vi "baseline_update.vi"(8 "current baseline phase":dbl, 9 "current baseline magnitude":dbl, 11 "Cluster in":T1={"Magnitude meas."=[], "Phase meas."=[], "Shift meas."=[], "cw"=TRUE, "projections per image"=0, "ramp-up readouts"=0, "current sense type"="", "Number of pulses per image"=0, "Rotation enabled"=TRUE, "Rotary position"=[], "Baseline magnitude"=0.0, "Baseline phase"=0.0, "Wait readouts"=0, "Shift waveform type"="", "Shift enabled"=TRUE, "Time domain data"=[], "Motor pulse duration"=0.0, "Shift start"=0.0, "Shift stop"=0.0, "Notes"="", "Reconstructed image"=bytes[0], "Rotary encoder type"="", "Image start"=timestamp(0 s since 1904-01-01), "Image stop"=timestamp(0 s since 1904-01-01), "readouts per projection"=0, "Recon enabled"=FALSE, "Bidirectional shift"=FALSE, "Imager mode"="", "Shift delay"=0.0, "Shift frequency"=0.0, "Image time (calc)"=0.0, "Initial encoder position"=0.0, "Recon data"=[], "Trigger line values"=[], "Bed position"=0.0, "Sample image"=bytes[0], "Patch amplitude"=0.0, "Patch frequency"=0.0, "Patch phase"=0.0}) -> (0 "new baseline phase":dbl format="%0.5f", 1 "new baseline magnitude":dbl format="%0.3p")   [LabVIEW 2019]
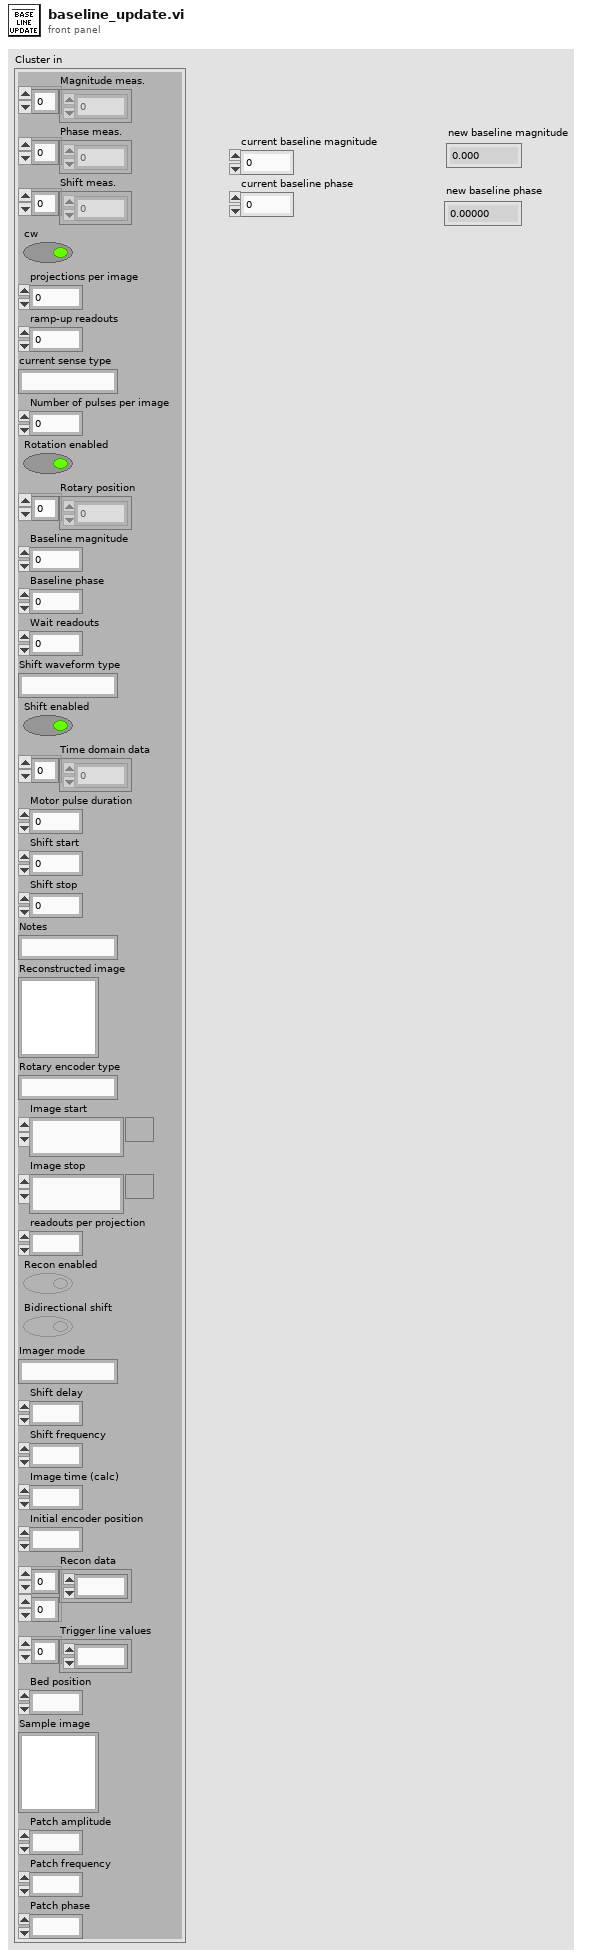
[diagram p1: front panel]
types:
  T1 = cluster{"Magnitude meas.":dbl[], "Phase meas.":dbl[], "Shift meas.":dbl[], "cw":bool, "projections per image":i32, "ramp-up readouts":i32, "current sense type":string, "Number of pulses per image":i32, "Rotation enabled":bool, "Rotary position":dbl[], "Baseline magnitude":dbl, "Baseline phase":dbl, "Wait readouts":i32, "Shift waveform type":string, "Shift enabled":bool, "Time domain data":dbl[], "Motor pulse duration":dbl, "Shift start":dbl, "Shift stop":dbl, "Notes":string, "Reconstructed image":picture, "Rotary encoder type":string, "Image start":timestamp, "Image stop":timestamp, "readouts per projection":i32, "Recon enabled":bool, "Bidirectional shift":bool, "Imager mode":string, "Shift delay":dbl, "Shift frequency":dbl, "Image time (calc)":dbl, "Initial encoder position":dbl, "Recon data":dbl[][], "Trigger line values":i32[], "Bed position":dbl, "Sample image":picture, "Patch amplitude":dbl, "Patch frequency":dbl, "Patch phase":dbl}
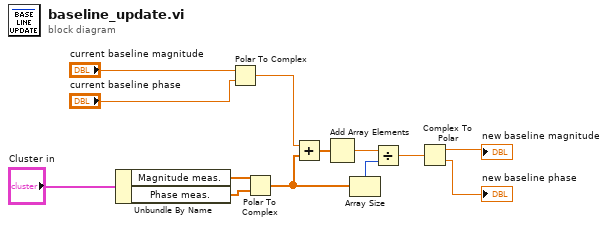
[diagram p0: block diagram]
diagram:
  n1 = Unbundle By Name("Cluster in") -> ("Magnitude meas."=w7:dbl[], "Phase meas."=w6:dbl[])
  n2 = Polar To Complex(1:"current baseline phase", 2:"current baseline magnitude") -> (0:w13:cdb)
  n3 = Polar To Complex(1:w6, 2:w7) -> (0:w11:cdb[])
  n4 = Add(x=w13, y=w11) -> (x+y=w12:cdb[])
  n5 = Add Array Elements(numeric array=w12) -> (sum=w10:cdb)
  n6 = Array Size(array=w11) -> (size(s)=w9:i32)
  n7 = Divide(x=w10, y=w9) -> (x/y=w8:cdb)
  n8 = Complex To Polar(r * e^(i*theta)=w8) -> (r=→"new baseline magnitude":dbl, theta=→"new baseline phase":dbl)
